vi "TP 3.1 1.vi"() -> ()   [LabVIEW 2013]
panel:
  in  "Stop":bool
  out "Waveform Graph":dbl[][](graph)
  in  "Amplitud":dbl=6.0
  in  "Frecuencia":dbl=10.0
  in  "Muestras por segundo":dbl=50.0
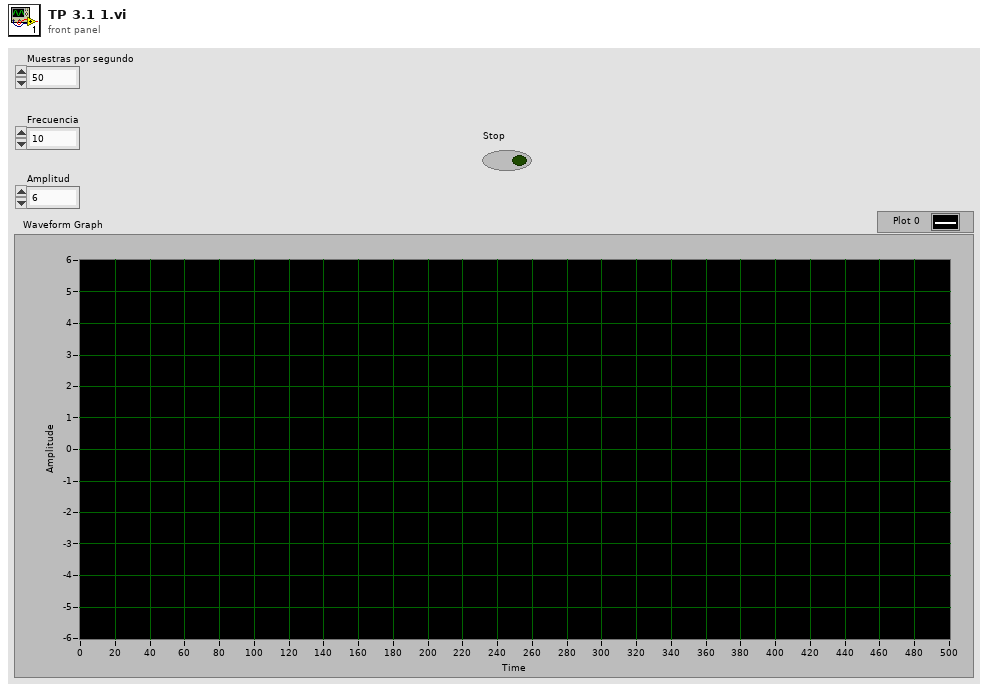
[diagram p1: front panel]
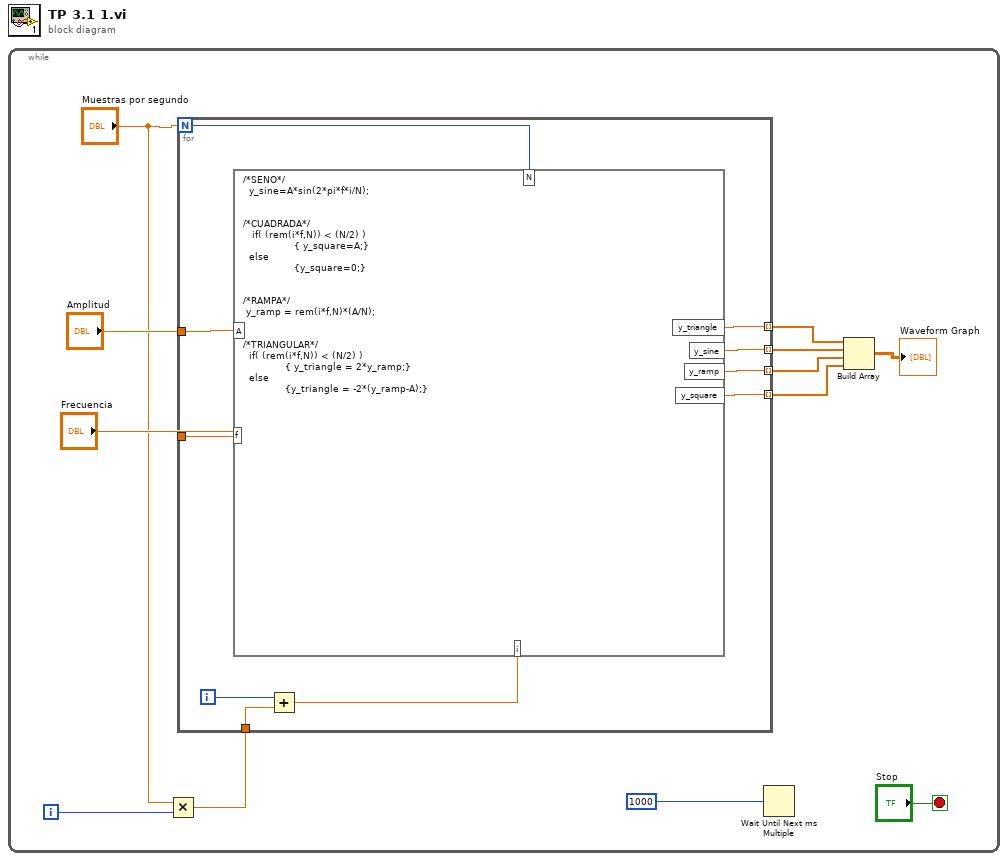
[diagram p0: block diagram]
diagram:
  n1 = while {
    i -> [w10]
    stop <- "Stop" stop-if-true
    n2 = Multiply(x="Muestras por segundo", y=w10) -> (x*y=w9:dbl)
    n3 = for {
      N: "Muestras por segundo" -> [w21]
      tunnel: "Frecuencia" -> [w13]
      tunnel: [w22] -> w7 mode=indexing
      tunnel: w9 -> [w14]
      tunnel: [w19] -> w3 mode=indexing
      tunnel: [w18] -> w2 mode=indexing
      tunnel: [w17] -> w1 mode=indexing
      tunnel: "Amplitud" -> [w16]
      i -> [w15]
      n4 = Add(x=w15, y=w14) -> (x+y=w20:dbl)
      n5 = formula code="/*SENO*/\n  y_sine=A*sin(2*pi*f*i/N);\n\n\n/*CUADRADA*/\n   if( (rem(i*f,N)) < (N/2) )\n                 { y_square=A;}\n  else\n                 {y_square=0;}\n\n\n/*RAMPA*/\n y_ramp = rem(i*f,N)*(A/N);\n\n\n/*TRIANGULAR*/\n  if( (rem(i*f,N)) < (N/2) )\n              { y_triangle = 2*y_ramp;}\n  else\n              {y_triangle = -2*(y_ramp-A);}"("A"=w16, "N"=w21, "i"=w20, "f"=w13) -> ("y_sine"=w22:dbl, "y_ramp"=w18:dbl, "y_square"=w17:dbl, "y_triangle"=w19:dbl)
    }
    n6 = Wait Until Next ms Multiple(millisecond multiple=u32 1000) -> ()  [unwired: 1 out]
    n7 = Build Array(w3, w7, w2, w1) -> (→"Waveform Graph":dbl[][])
  }
